vi "Teach Window Activation and Click Position.vi"() -> ()   [LabVIEW 2022 SP3]
panel:
  out "Message":string
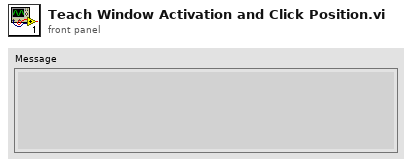
[diagram p1: front panel]
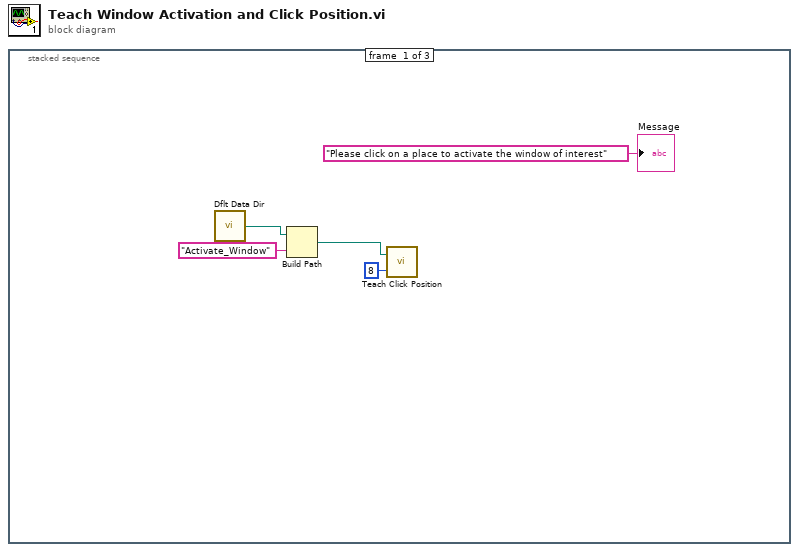
[diagram p0: block diagram]
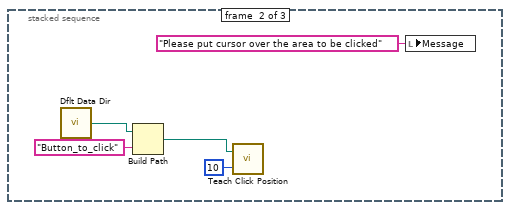
[diagram p2: hidden frame]
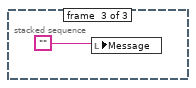
[diagram p3: hidden frame]
diagram:
  n1 = stacked-sequence {
    frame #0 {
      n2 = call <vilib>:"Dflt Data Dir.vi"() -> ("App:Default Data Directory"=w5:path)
      n3 = Build Path(base path=w5, name or relative path="Activate_Window") -> (appended path=w3:path)
      n4 = call "Teach Click Position.vi"("Wait time (s)"=8, "Click position file path"=w3) -> ()  [unwired: 2 out]
      "Message" <- "Please click on a place to activate the window of interest" ("Message")
    }
    frame #1 {
      n5 = call <vilib>:"Dflt Data Dir.vi"() -> ("App:Default Data Directory"=w10:path)
      n6 = Build Path(base path=w10, name or relative path="Button_to_click") -> (appended path=w8:path)
      n7 = call "Teach Click Position.vi"("Wait time (s)"=10, "Click position file path"=w8) -> ()  [unwired: 2 out]
      n8 = local write "Message"("Please put cursor over the area to be clicked" ("Message")) -> ()
    }
    frame #2 {
      n9 = local write "Message"("") -> ()
    }
  }
